vi "serial-csv-to-string-array.vi"(8 "error in (no error)":errorcluster, 11 "VISA Refnum in":refnum<visa-resource-name>) -> (0 "error out":errorcluster, 1 "timestamp":i32, 2 "data string array":string[](array[string]), 3 "VISA Refnum out":refnum<visa-resource-name>, 4 "Bytes Returned":u32, 5 "read buffer":string)   [LabVIEW 2021]
uses:
  <vilib>/regexp/Match Regular Expression.xnode
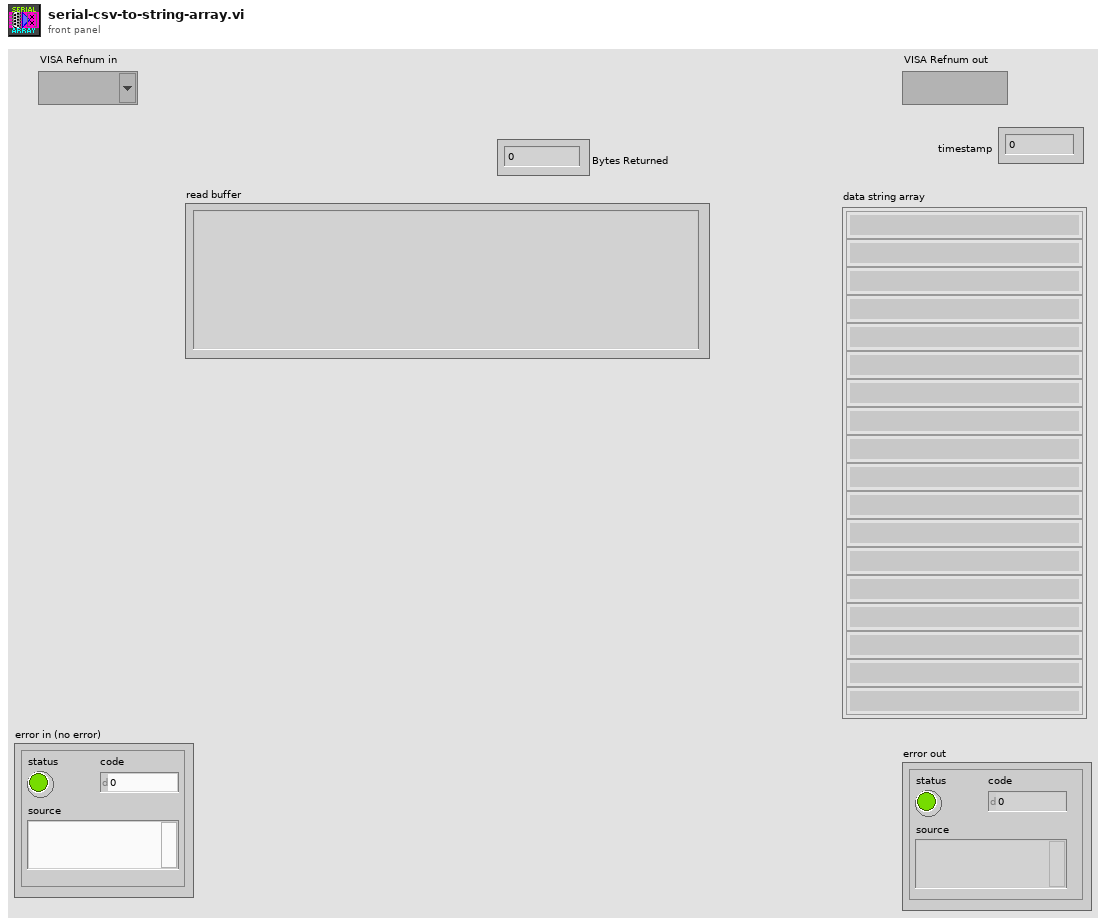
[diagram p1: front panel]
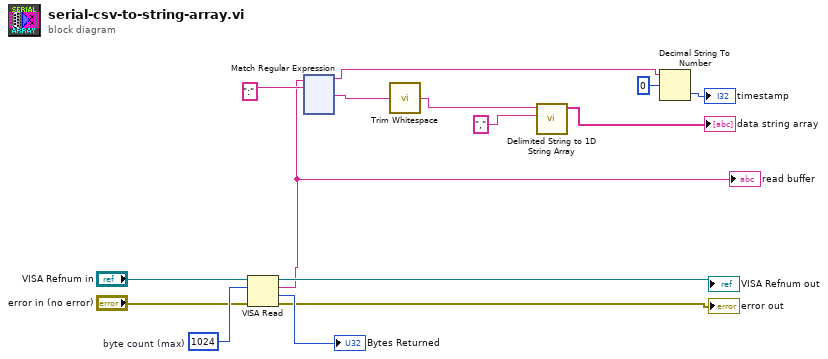
[diagram p0: block diagram]
diagram:
  w6 = u32 1024  # byte count (max)
  n1 = VISA Read(VISA resource name="VISA Refnum in", byte count=w6, error in (no error)="error in (no error)") -> (VISA resource name out=→"VISA Refnum out":refnum<visa-resource-name>, read buffer=w2:string, return count=→"Bytes Returned":u32, error out=→"error out":errorcluster)
  "read buffer" <- w2
  n2 = xnode "Match Regular Expression"("input string"=w2, "regular expression"=":" ("delimiter")) -> ("before match"=w10:string, "after match"=w12:string)  [unwired: 4 in, 3 out]
  n3 = call <vilib>:"Trim Whitespace.vi"("string"=w12) -> ("trimmed string"=w13:string)  [unwired: 1 in]
  n4 = call <vilib>:"Delimited String to 1D String Array.vi"("delimiter"=",", "delimited string"=w13) -> ("string array"=→"data string array":string[])  [unwired: 9 in]
  n5 = Decimal String To Number(string=w10, offset=0) -> (number=→"timestamp":i32)  [unwired: 1 in, 1 out]
